vi "Create RFFE Read Waveform_wo_SetID.vi"(0 "Data":T1 {"Register" format="%.0x"; "Slave Address" max=15 format="%.0x"}, 1 "Ext_Read_Num_Reg":u8, 2 "Readback Speed":enum16{"Full Speed", "Half Speed"}(ring), 5 "Configuratation":T2={"Samples to Allocate"=10000, "Oversample Factor"=1, "Clock Channel"=enum."0", "Data Channel"=enum."1"} {"Oversample Factor" min=1 max=254; "Samples to Allocate" min=1}, 11 "error in (no error)":errorcluster) -> (6 "Waveform Graph":digitalwaveform(graph), 15 "error out":errorcluster)   [LabVIEW 2013]
uses:
  Ctrls/Configuration.ctl
  Ctrls/ClockDataChannels.ctl
  Ctrls/RegReadWrite.ctl
  Ctrls/ExtendedRegReadWrite.ctl
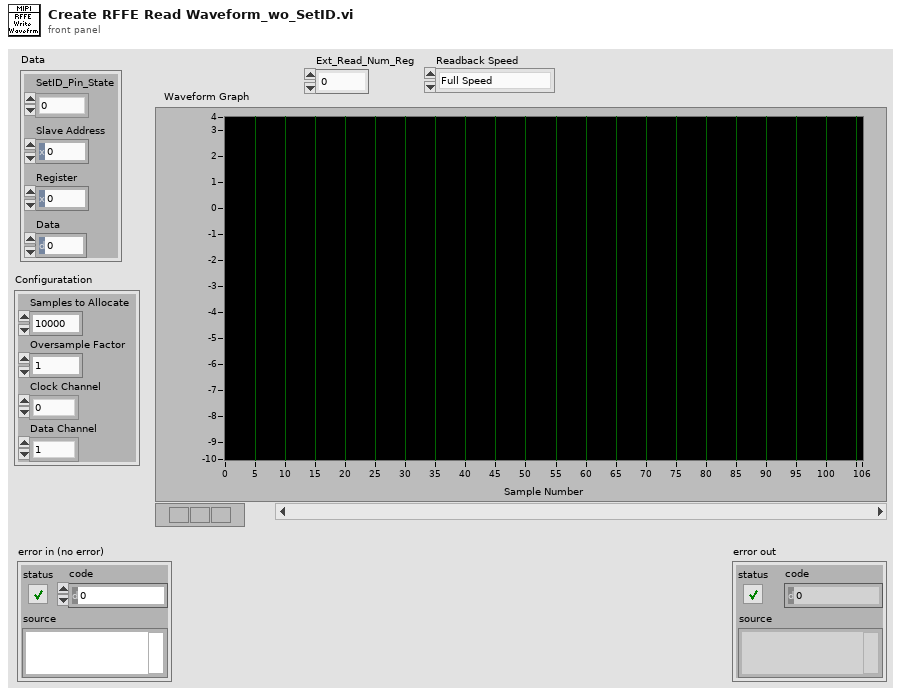
[diagram p1: front panel]
types:
  T1 = typedef "RegReadWrite.ctl" = cluster{"Slave Address":u8, "Register":u8, "Data":u8, "SetID_Pin_State":enum16{"0", "1", "Z"}}
  T2 = typedef "Configuration.ctl" = cluster{"Samples to Allocate":i32, "Oversample Factor":u8, "Clock Channel":T3, "Data Channel":T3}
  T3 = typedef "ClockDataChannels.ctl" = enum16{"0", "1"}
  T4 = typedef "RFFE_Data.ctl" = cluster{"Clock Channel":T3, "Data Channel":T3, "Oversample Factor":u8, "Zero Array":u8[], "One Array":u8[], "Z Array ":u8[], "H Array":u8[], "L Array":u8[], "X Array":u8[], "Toggle (high to low)":u8[]}
  T5 = typedef "ExtendedRegReadWrite.ctl" = cluster{"Slave Address":u8, "Register":u8, "Data":u8[]}
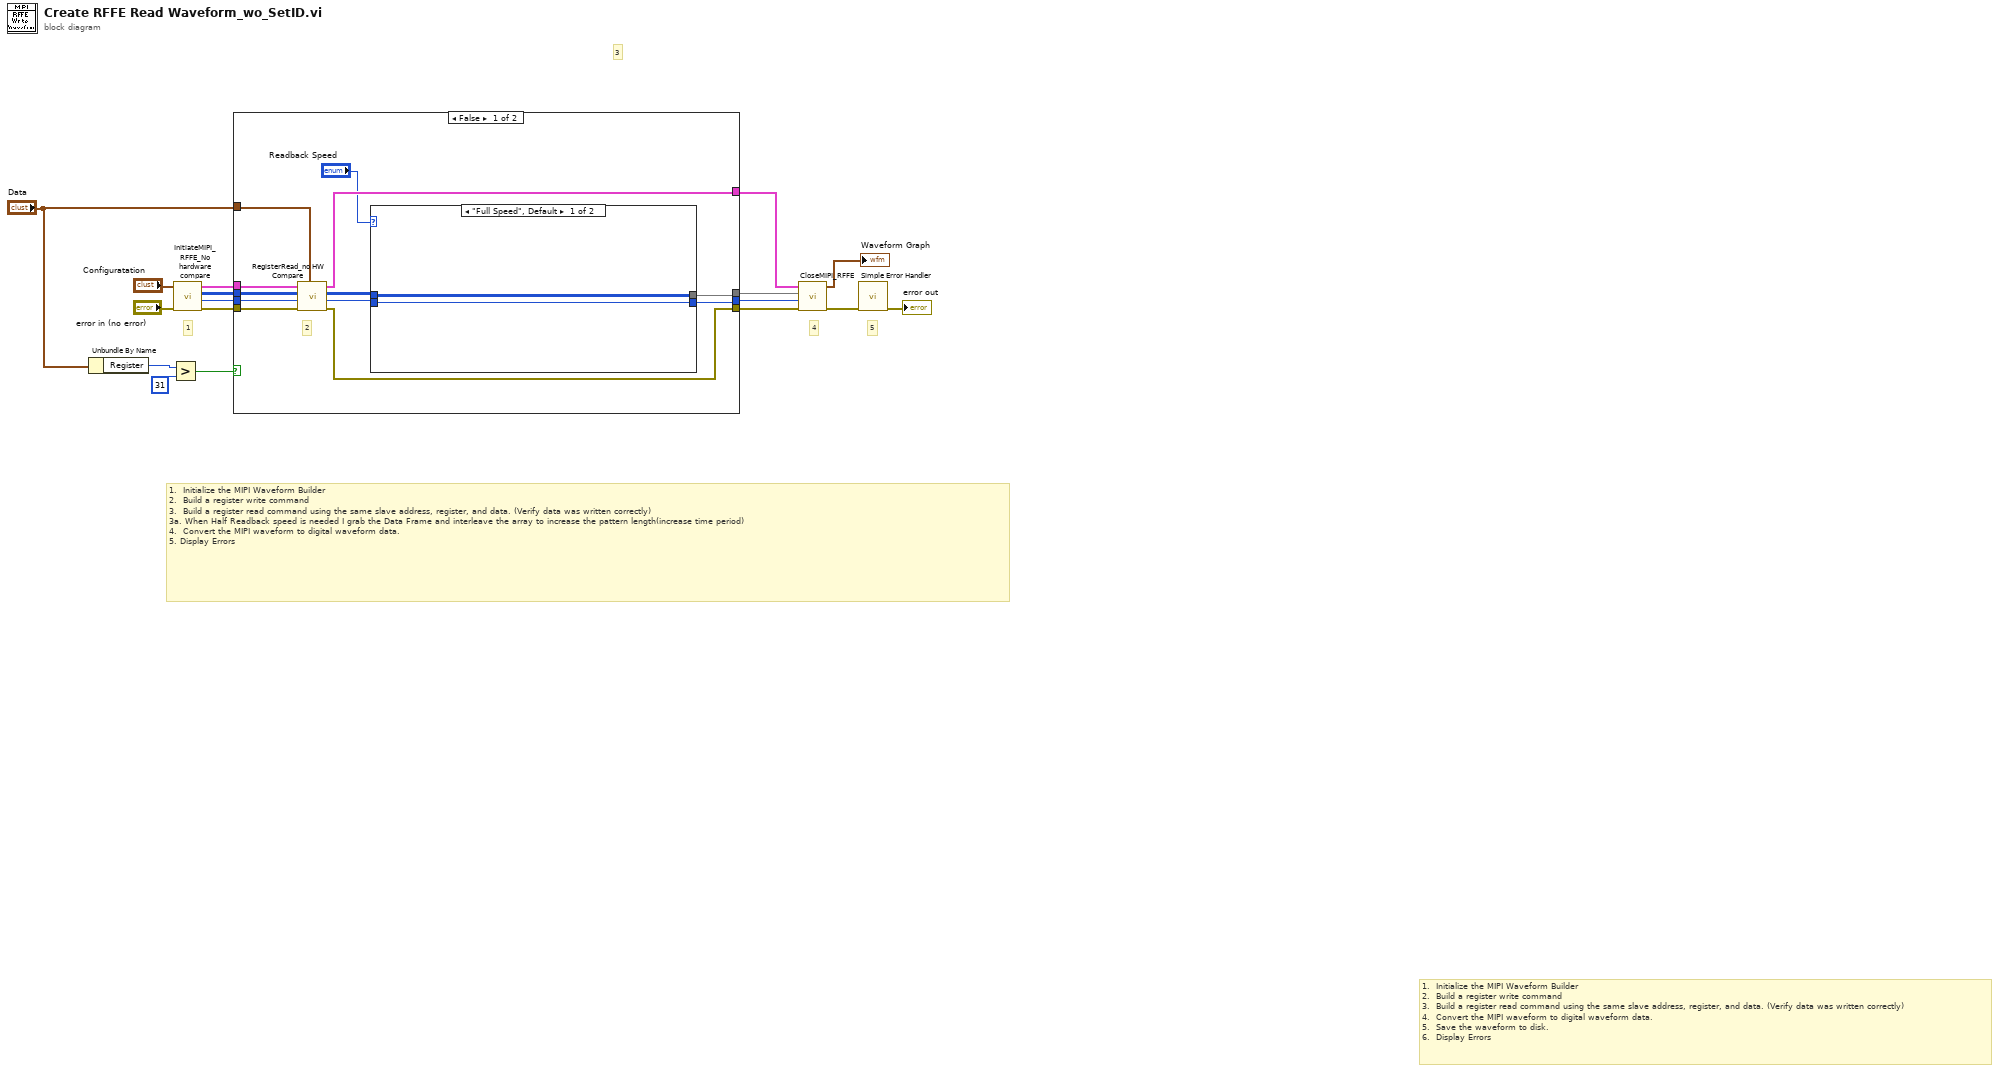
[diagram p0: block diagram]
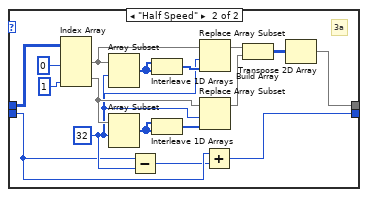
[diagram p2: hidden frame]
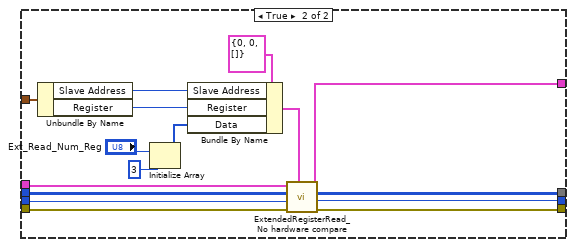
[diagram p3: hidden frame]
diagram:
  # "3"
  # "1.  Initialize the MIPI Waveform Builder\n2.  Build a register write command\n3.  Build a register read command using the same slave address, register, and data. (Verify data was written correctly)\n3a. When Half Readback speed is needed I grab the Data Frame and interleave the array to increase the pattern length(increase time period)\n4.  Convert the MIPI waveform to digital waveform data.\n5. Display Errors"
  # "5"
  # "1.  Initialize the MIPI Waveform Builder\n2.  Build a register write command\n3.  Build a register read command using the same slave address, register, and data. (Verify data was written correctly)\n4.  Convert the MIPI waveform to digital waveform data.\n5.  Save the waveform to disk.\n6.  Display Errors"
  # "4"
  # "1"
  n1 = Unbundle By Name("Data") -> ("Register"=w5:u8)
  n2 = Greater?(x=w5, y=u8 31) -> (0:w3:bool)
  n3 = call "InitiateMIPI_RFFE_No hardware compare.vi"("error in (no error)"="error in (no error)", "Configuratation In"="Configuratation") -> ("error out"=w10:errorcluster, "Number of Samples Out"=w11:i32, "Data Array"=w12:u8[][], "RFFE_Data"=w13:T4)  [unwired: 6 in]
  n4 = case shown="False" w3 {
    tunnel: w13 -> [w29 w63]
    tunnel: w12 -> [w28 w62]
    tunnel: w11 -> [w27 w61]
    tunnel: w10 -> [w26 w64]
    tunnel: [w25 w55] -> w9
    tunnel: [w24 w52] -> w8
    tunnel: [w21 w54] -> w7
    tunnel: [w19 w53] -> w6
    tunnel: "Data" -> [w18 w60]
    frame False {
      # "2"
      n5 = call "RegisterRead_no HW Compare.vi"("Register Read/Write"=w18, "error in (no error)"=w26, "Number of Samples In"=w27, "Data Array"=w28, "RFFE_Data In"=w29) -> ("error out"=w25:errorcluster, "Number of Samples Out out"=w20:i32, "Data Array Out"=w22:u8[][], "RFFE_Data Out"=w24:T4)  [unwired: 2 in, 1 out]
      n6 = case shown="\"Full Speed\", Default" "Readback Speed" {
        tunnel: w22 -> [w31 w37]
        tunnel: [w31 w36] -> w21
        tunnel: w20 -> [w30 w34]
        tunnel: [w30 w32] -> w19
        frame "Full Speed", Default {
        }
        frame "Half Speed" {
          w35 = 32 ("index")
          # "3a"
          n7 = Index Array(array=w37, index (col) #1=0 ("index (row)"), index (col) #2=1 ("index (row)")) -> (element #1=w42:u8[], element #2=w47:u8[])  [unwired: 2 in]
          n8 = Array Subset(array=w42, index=w35) -> (w38:u8[])  [unwired: 1 in]
          n9 = Array Subset(array=w47, index=w35) -> (w39:u8[])  [unwired: 1 in]
          n10 = Subtract(x=w34, y=w35) -> (x-y=w33:i32)
          n11 = Interleave 1D Arrays(w38, w38) -> (w48:u8[])
          n12 = Interleave 1D Arrays(w39, w39) -> (w43:u8[])
          n13 = Replace Array Subset(array=w42, new element=w48, index=w35) -> (w44:u8[])
          n14 = Replace Array Subset(array=w47, new element=w43, index=w35) -> (w46:u8[])
          n15 = Add(x=w34, y=w33) -> (x+y=w32:i32)
          n16 = Build Array(w44, w46) -> (w45:u8[][])
          n17 = Transpose 2D Array(2D array=w45) -> (transposed array=w36:u8[][])
        }
      }
    }
    frame True {
      n18 = Unbundle By Name(w60) -> ("Slave Address"=w58:u8, "Register"=w59:u8)
      n19 = Initialize Array("Ext_Read_Num_Reg", 3 ("dimension size")) -> (w49:u8[])
      n20 = Bundle By Name(cluster=T5 {"Slave Address"=0, "Register"=0, "Data"=[]} ("Extended Read/Write"), "Slave Address"=w58, "Register"=w59, "Data"=w49) -> (w56:T5)
      n21 = call "ExtendedRegisterRead_No hardware compare.vi"("Extended Read/Write"=w56, "error in (no error)"=w64, "Number of Samples In"=w61, "Data Array"=w62, "RFFE_Data In"=w63) -> ("error out"=w55:errorcluster, "Number of Samples Out out"=w53:i32, "Data Array Out"=w54:u8[][], "RFFE_Data Out"=w52:T4)  [unwired: 3 in]
    }
  }
  n22 = call "CloseMIPI_RFFE.vi"("error in (no error)"=w9, "Number of Samples"=w6, "Data Array"=w7, "RFFE_Data"=w8) -> ("error out"=w16:errorcluster, "Digital Waveform"=→"Waveform Graph":digitalwaveform)  [unwired: 6 in]
  n23 = call <vilib>:"Simple Error Handler.vi"("error in (no error)"=w16) -> ("error out"=→"error out":errorcluster)  [unwired: 4 in, 4 out]
